vi "Read EDVR Pool.vi"(11 "Template in":refnum<class "Template.lvclass">) -> (3 "DVR Pool":refnum<queue>)   [LabVIEW 2020, in "Template.lvlib" / "Template.lvclass"]
doc: "Returns the DVR Pool queue reference"
uses:
  Template.lvclass
  Template.lvclass/Template.ctl
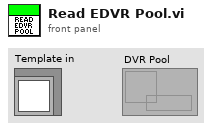
[diagram p1: front panel]
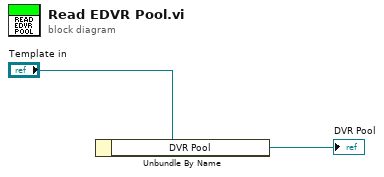
[diagram p0: block diagram]
diagram:
  n1 = Unbundle By Name("Template in") -> ("DVR Pool"=→"DVR Pool":refnum<queue>)
